vi "4 memory dds 1SPC.vi"(0 "new PDW in":bool, 1 "stop this pulse":bool, 5 "free DDS before me?":bool, 7 "run":bool=TRUE, 9 "pdw in":T3 {"frequency shift" format="%#_12f"}, 11 "referenses":T2={"clock x2"="IO Socket\\Data Clock 2x", "Memory In"="pulse on memory", "Memory In 2"="pulse on memory", "Memory In 3"="pulse on memory", "Memory In 4"="pulse on memory"}) -> (4 "output cluster":T1, 6 "have free DDS":bool, 10 "state of every DDS":bool[](array[boolean]), 15 "output valid":bool)   [LabVIEW 2021]
doc: "transmit pulse with one free DDS inside.\nmust have no DDS before him (the distribute is to give the lowest mun DDS the pulse)"
uses:
  pulse_tx_vis/pdw.ctl
  pulse_tx_vis/CTL/mode_type.ctl
  <instrlib>/_niInstr/DSP/v1/Shared/Public/IQ Data.ctl
  <instrlib>/_niInstr/DSP/v1/Shared/niInstr DSP v1 Shared.lvlib
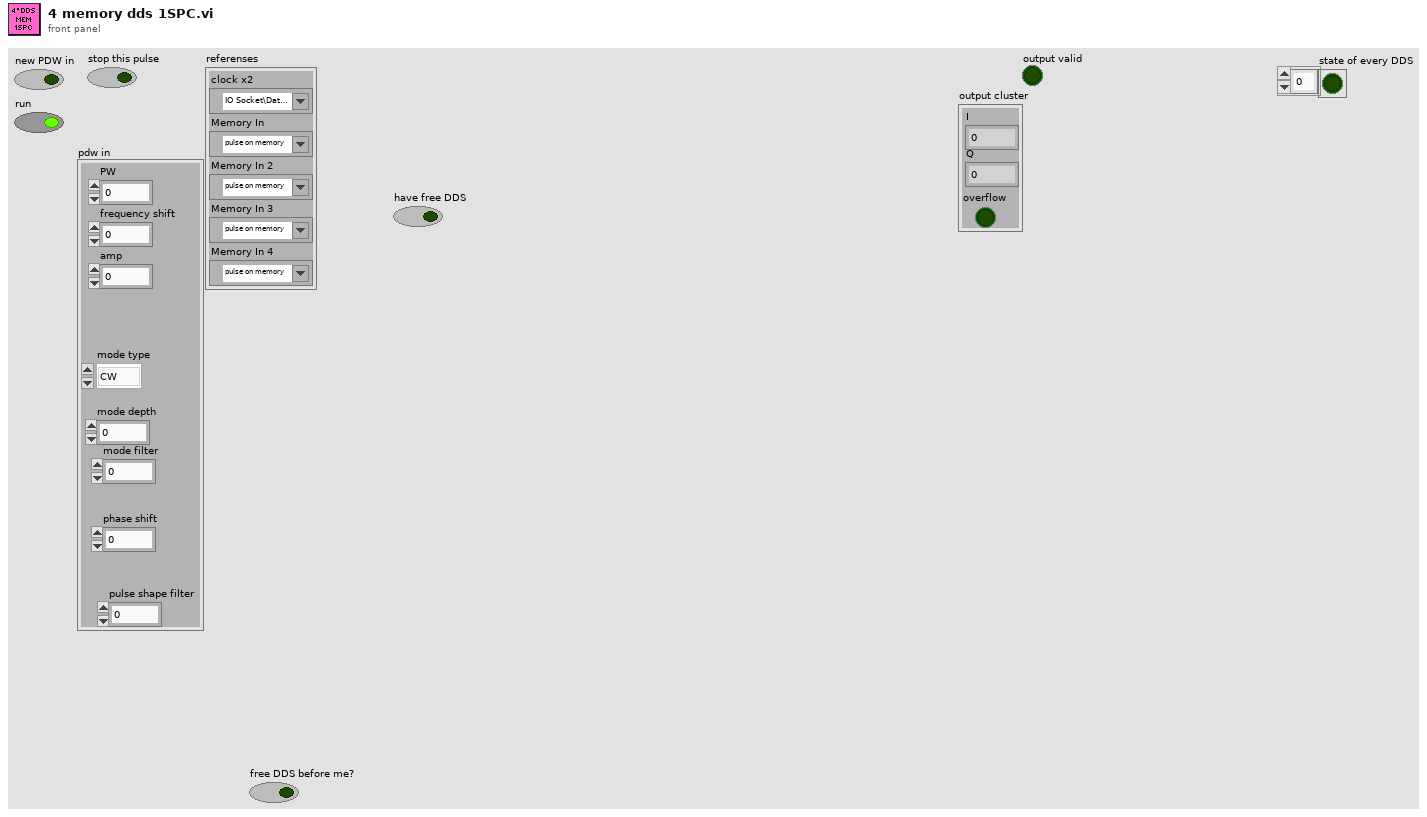
[diagram p1: front panel]
types:
  T1 = typedef "niInstr DSP v1 Shared.lvlib/IQ Data.ctl" = cluster{"I":fxp<+/-,18,1>, "Q":fxp<+/-,18,1>, "overflow":bool}
  T2 = cluster{"clock x2":refnum<k21>, "Memory In":refnum<k21>, "Memory In 2":refnum<k21>, "Memory In 3":refnum<k21>, "Memory In 4":refnum<k21>}
  T3 = typedef "pdw.ctl" = cluster{"PW":u32, "frequency shift":fxp<+/-,48,0>, "amp":fxp<+/-,18,1>, "mode type":T4, "mode depth":u32, "mode filter":u8, "phase shift":fxp<+/-,16,1>, "pulse shape filter":u8}
  T4 = typedef "mode_type.ctl" = enum8{"CW", "from memory 1", "NC - cw", "LFM", "BPSK", "QPSK"}
  T5 = cluster{"clock x2":refnum<k21>, "Memory In":refnum<k21>}
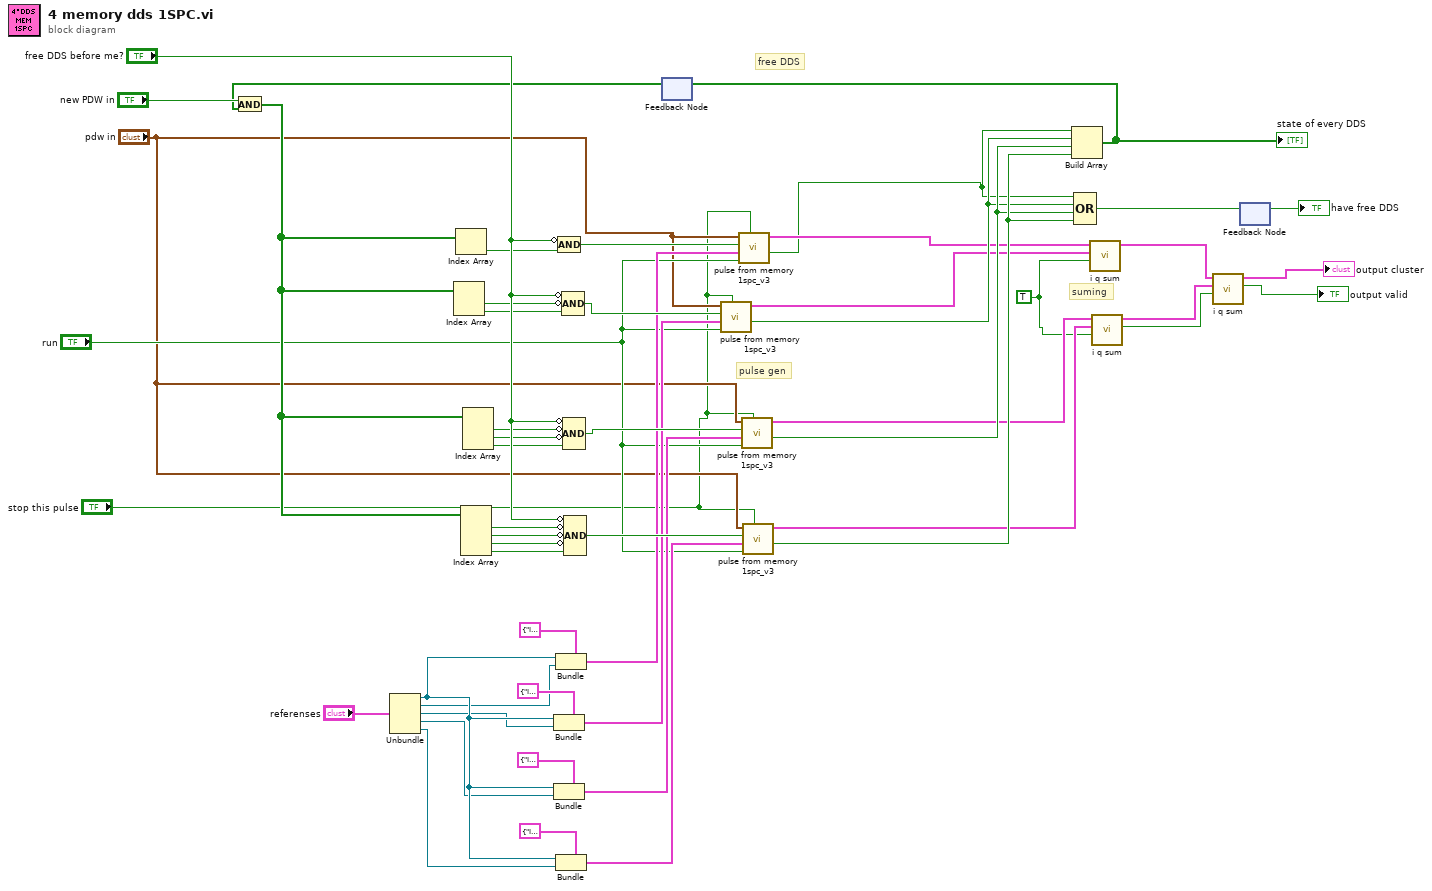
[diagram p0: block diagram]
diagram:
  w19 = TRUE ("input valid")
  # "free DDS"
  # "suming"
  # "pulse gen"
  n1 = Unbundle("referenses") -> ("clock x2"=w13:refnum<k21>, "Memory In"=w9:refnum<k21>, "Memory In 2"=w10:refnum<k21>, "Memory In 3"=w11:refnum<k21>, "Memory In 4"=w12:refnum<k21>)
  n2 = Bundle(cluster=T5 {"clock x2"="IO Socket\\Data Clock 2x", "Memory In"="pulse on memory"} ("referenses"), "clock x2"=w13, "Memory In"=w10) -> (w7:T5)
  n3 = Bundle(cluster=T5 {"clock x2"="IO Socket\\Data Clock 2x", "Memory In"="pulse on memory"} ("referenses"), "clock x2"=w13, "Memory In"=w11) -> (w6:T5)
  n4 = Bundle(cluster=T5 {"clock x2"="IO Socket\\Data Clock 2x", "Memory In"="pulse on memory"} ("referenses"), "clock x2"=w13, "Memory In"=w9) -> (w8:T5)
  n5 = Bundle(cluster=T5 {"clock x2"="IO Socket\\Data Clock 2x", "Memory In"="pulse on memory"} ("referenses"), "clock x2"=w13, "Memory In"=w12) -> (w5:T5)
  n6 = feedback #1() -> (w28:bool[])  [unwired: 1 in]
  n7 = And(x="new PDW in", y=w28) -> (x .and. y?=w27:bool[])
  n8 = Index Array(array=w27) -> (element #1=w39:bool, element #2=w37:bool)  [unwired: 2 in]
  n9 = Index Array(array=w27) -> (element=w35:bool)  [unwired: 1 in]
  n10 = Index Array(array=w27) -> (element #1=w47:bool, element #2=w46:bool, element #3=w45:bool, element #4=w44:bool)  [unwired: 4 in]
  n11 = Index Array(array=w27) -> (element #1=w43:bool, element #2=w42:bool, element #3=w41:bool)  [unwired: 3 in]
  n12 = Compound Arithmetic op=AND(invert "free DDS before me?", w35) -> (w36:bool)
  n13 = Compound Arithmetic op=AND(invert "free DDS before me?", invert w39, w37) -> (w38:bool)
  n14 = Compound Arithmetic op=AND(invert "free DDS before me?", invert w43, invert w42, w41) -> (w40:bool)
  n15 = Compound Arithmetic op=AND(invert "free DDS before me?", invert w47, invert w46, invert w45, w44) -> (w48:bool)
  n16 = call "pulse from memory 1spc_v3.vi"("stop this pulse"="stop this pulse", "run"="run", "referenses"=w7, "start this pulse"=w38, "PDW"="pdw in") -> ("free DDS"=w49:bool, "IQ out"=w32:T1)  [unwired: 4 in, 1 out]
  n17 = call "pulse from memory 1spc_v3.vi"("stop this pulse"="stop this pulse", "run"="run", "referenses"=w8, "start this pulse"=w36, "PDW"="pdw in") -> ("free DDS"=w20:bool, "IQ out"=w31:T1)  [unwired: 4 in, 1 out]
  n18 = call "pulse from memory 1spc_v3.vi"("stop this pulse"="stop this pulse", "run"="run", "referenses"=w6, "start this pulse"=w40, "PDW"="pdw in") -> ("free DDS"=w50:bool, "IQ out"=w33:T1)  [unwired: 4 in, 1 out]
  n19 = call "pulse from memory 1spc_v3.vi"("stop this pulse"="stop this pulse", "run"="run", "referenses"=w5, "start this pulse"=w48, "PDW"="pdw in") -> ("free DDS"=w51:bool, "IQ out"=w34:T1)  [unwired: 4 in, 1 out]
  n20 = Build Array(w20, w49, w50, w51) -> (w30:bool[])
  "state of every DDS" <- w30
  n21 = feedback-in #1(w30) -> ()
  n22 = Compound Arithmetic op=OR(w20, w49, w50, w51) -> (w26:bool)
  n23 = call "i q sum.vi"("input valid"=w19, 10:"data in"=w32, 11:"data in"=w31) -> ("output cluster"=w24:T1)  [unwired: 7 in, 1 out]
  n24 = call "i q sum.vi"("input valid"=w19, 10:"data in"=w34, 11:"data in"=w33) -> ("output valid"=w22:bool, "output cluster"=w23:T1)  [unwired: 7 in]
  n25 = call "i q sum.vi"("input valid"=w22, 10:"data in"=w23, 11:"data in"=w24) -> ("output valid"=→"output valid":bool, "output cluster"=→"output cluster":T1)  [unwired: 7 in]
  n26 = feedback #2() -> (→"have free DDS":bool)  [unwired: 1 in]
  n27 = feedback-in #2(w26) -> ()
